vi "Timestamp_to_UTC.vi"(11 "Timestamp":timestamp format="%<%.6X\n%x>T") -> (2 "Timestamp (s)":dbl format="%#_8g", 3 "UTC Time":u64)   [LabVIEW 2020]
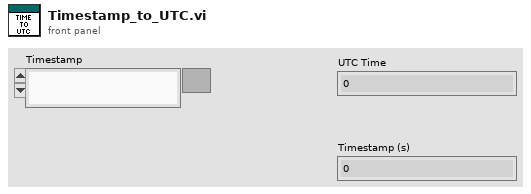
[diagram p1: front panel]
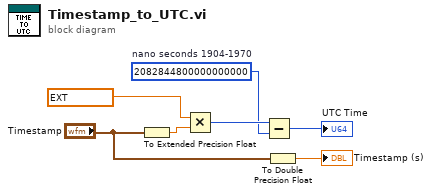
[diagram p0: block diagram]
diagram:
  w5 = u64 2082844800000000000  # nano seconds 1904-1970
  n1 = To Extended Precision Float(1:"Timestamp") -> (0:w7:ext)
  n2 = Multiply(x=ext 1000000000.0, y=w7) -> (x*y=w6:u64)
  n3 = Subtract(x=w6, y=w5) -> (x-y=→"UTC Time":u64)
  n4 = To Double Precision Float(number="Timestamp") -> (double precision float=→"Timestamp (s)":dbl)
